vi "RvsT Error Handler.vi"(7 "Restart on errors":bool, 8 "error in (no error)":errorcluster, 9 "Start measurement":refnum<user-event>, 10 "Stop measurement":refnum<user-event>, 11 "Log File Path":path) -> (0 "error out":errorcluster, 4 "Last Error":errorcluster)   [LabVIEW 2015]
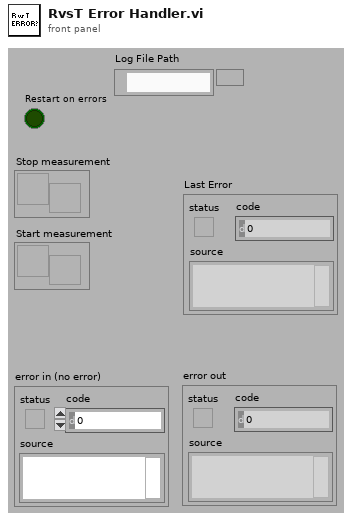
[diagram p1: front panel]
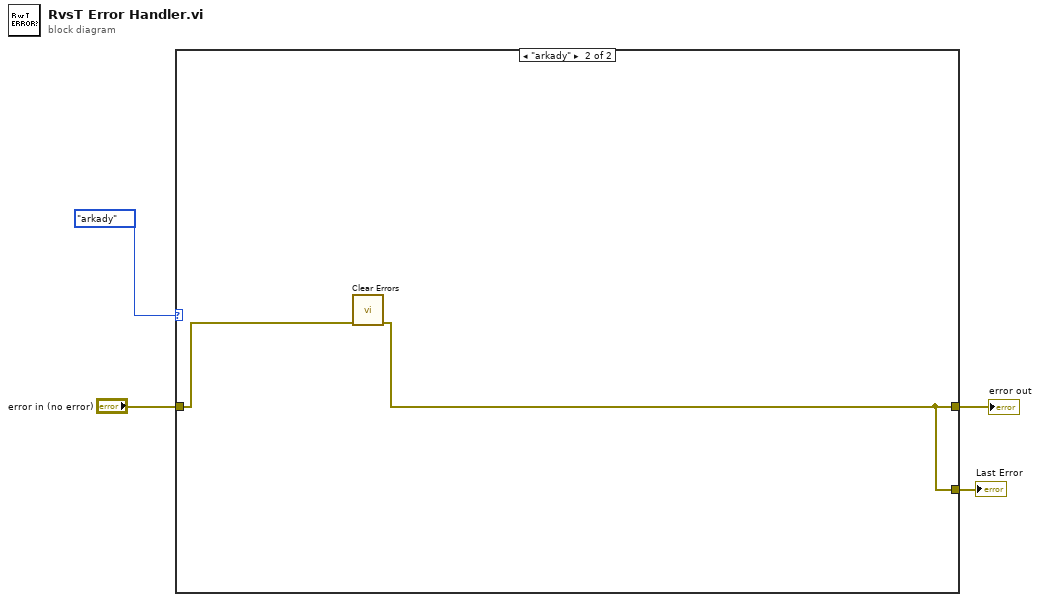
[diagram p0: block diagram]
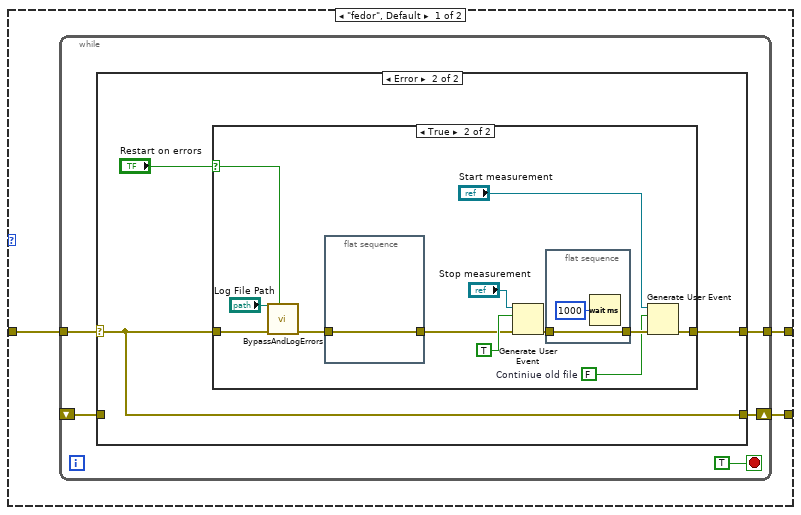
[diagram p2: hidden frame]
diagram:
  n1 = case shown="\"arkady\"" enum16{"fedor", "arkady"}."arkady" {
    tunnel: "error in (no error)" -> [w7 w35]
    tunnel: [w6 w34] -> w3
    tunnel: [w5 w34] -> w2
    frame "fedor", Default {
      n2 = while {
        tunnel: w7 -> [w12]
        tunnel: [w11] -> w6
        shift-right: [w10] -> w5
        shift-left: _ -> [w9]
        stop <- TRUE stop-if-true
        n3 = case shown="Error" w12 {
          selector: w12 -> [w14 w15]
          tunnel: [w14 w16] -> w11
          tunnel: [w13 w15] -> w10
          tunnel: w9 -> [w13 _]
          frame No Error {
          }
          frame Error {
            n4 = case shown="True" "Restart on errors" {
              selector: "Restart on errors" -> [_ w27]
              tunnel: w15 -> [w18 w26]
              tunnel: [w18 w24] -> w16
              frame False {
              }
              frame True {
                w19 = FALSE  # Continiue old file
                n5 = call "BypassAndLogErrors.vi"("Bypass Errors"=w27, "error in (no error)"=w26, "Log File Path"="Log File Path") -> ("error out"=w21:errorcluster)  [unwired: 8 out]
                n6 = flat-sequence {
                  tunnel: w21 -> [w31]
                  tunnel: [w31] -> w20
                  frame #0 {
                  }
                }
                n7 = Generate User Event(user event="Stop measurement", event data cluster=TRUE ("event data"), error in=w20) -> (error out=w23:errorcluster)  [unwired: 1 in, 1 out]
                n8 = flat-sequence {
                  tunnel: w23 -> [w33]
                  tunnel: [w33] -> w22
                  frame #0 {
                    n9 = Wait (ms)(milliseconds to wait=u32 1000) -> ()  [unwired: 1 out]
                  }
                }
                n10 = Generate User Event(user event="Start measurement", event data cluster=w19, error in=w22) -> (error out=w24:errorcluster)  [unwired: 1 in, 1 out]
              }
            }
          }
        }
      }
    }
    frame "arkady" {
      n11 = call <vilib>:"Clear Errors.vi"("error in (no error)"=w35) -> ("error out"=w34:errorcluster)  [unwired: 5 in, 1 out]
    }
  }
  "error out" <- w3
  "Last Error" <- w2
